vi "PD250 - PWM test_v2.vi"(8 "error in":errorcluster, 9 "Board Selector":T1, 10 "HMP VISA":refnum<visa-resource-name>, 11 "Control Board VISA":refnum<visa-resource-name>="ControlBoard") -> (0 "error out":errorcluster, 2 "Message OUT":string, 3 "Result (bool)":bool)   [LabVIEW 2022 SP3]
uses:
  Serial Board Com/Board Select.ctl
  HMP4000 Communication/HMP4040_ChannelControlAutomatic.ctl
  <vilib>/DAQmx/read.llb/DAQmx Read (Analog 1D Wfm NChan NSamp).vi
  <vilib>/DAQmx/miscellaneous.llb/DAQmx Fill In Error Info.vi
panel:
  out "Duty Cycle VISA Write":string[](array[string])
  out "ControlBoard OUT":refnum<visa-resource-name>
  in  "Message IN":string=" "
  out "Analysis Leg":i32
  out "Waveforms":T2
  out "Active Leg":i32
  out "Result (color)":u32(colorbox)
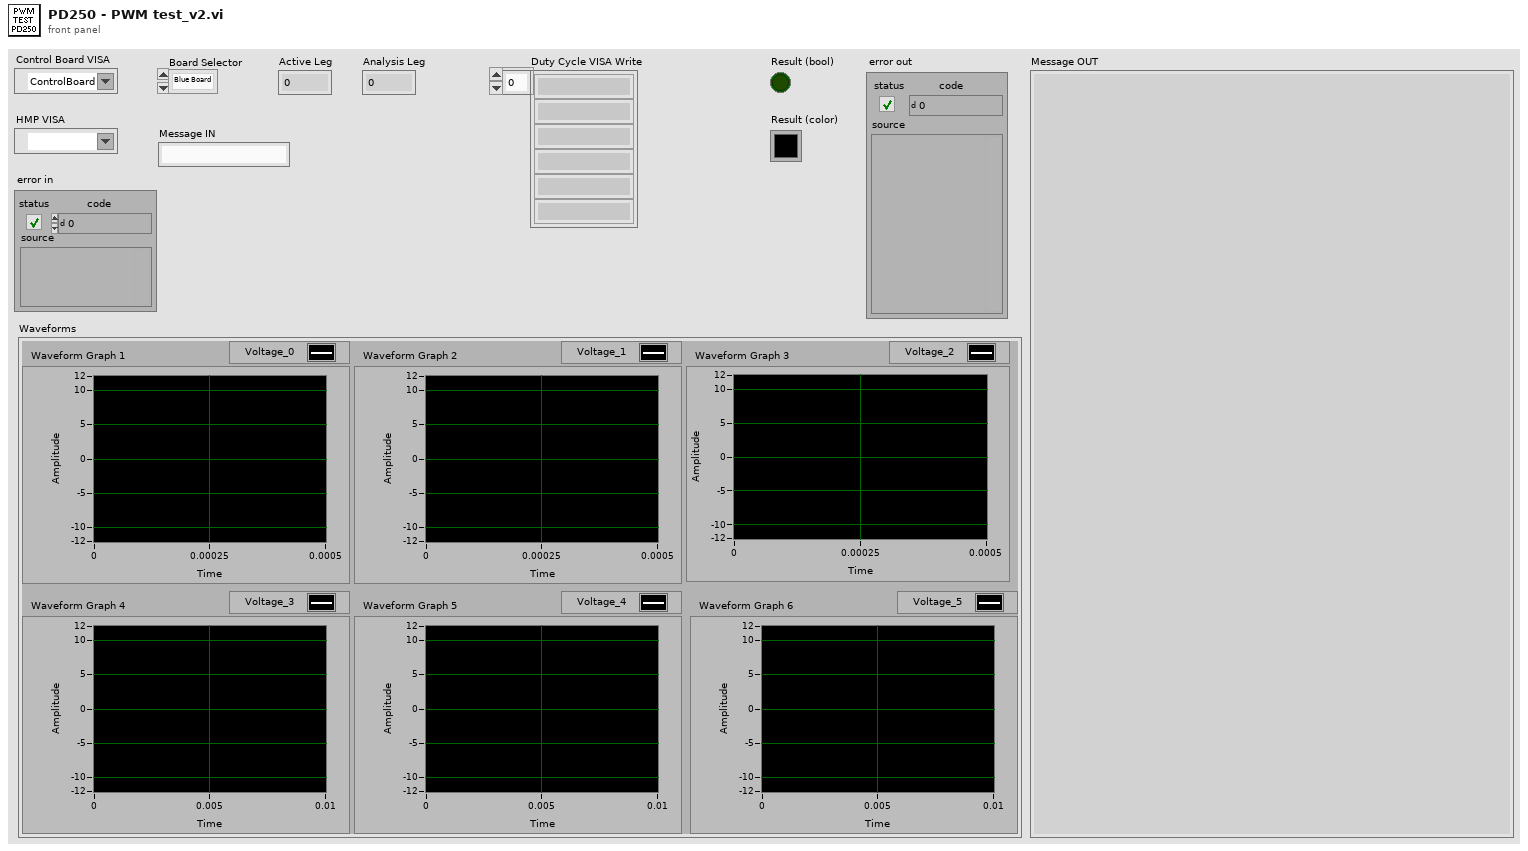
[diagram p1: front panel]
types:
  T1 = typedef "Board Select.ctl" = enum16{"Blue Board", "Green Board"}
  T2 = cluster{"Waveform Graph 1":waveform(dbl), "Waveform Graph 2":waveform(dbl), "Waveform Graph 3":waveform(dbl), "Waveform Graph 4":waveform(dbl), "Waveform Graph 5":waveform(dbl), "Waveform Graph 6":waveform(dbl)}
  T3 = typedef "HMP4040_ChannelControlAutomatic.ctl" = enum16{"Off", "Control Power", "HMP2020 Control + DC32V", "HMP2020 Control + DC8V", "HMP4040 Control + DC32V", "HMP4040 Control +DC8V", "HMP4040 Ch2 24V 4A"}
  T4 = cluster{"data[0]":waveform(dbl), "data[1]":waveform(dbl), "data[2]":waveform(dbl), "data[3]":waveform(dbl), "data[4]":waveform(dbl), "data[5]":waveform(dbl)}
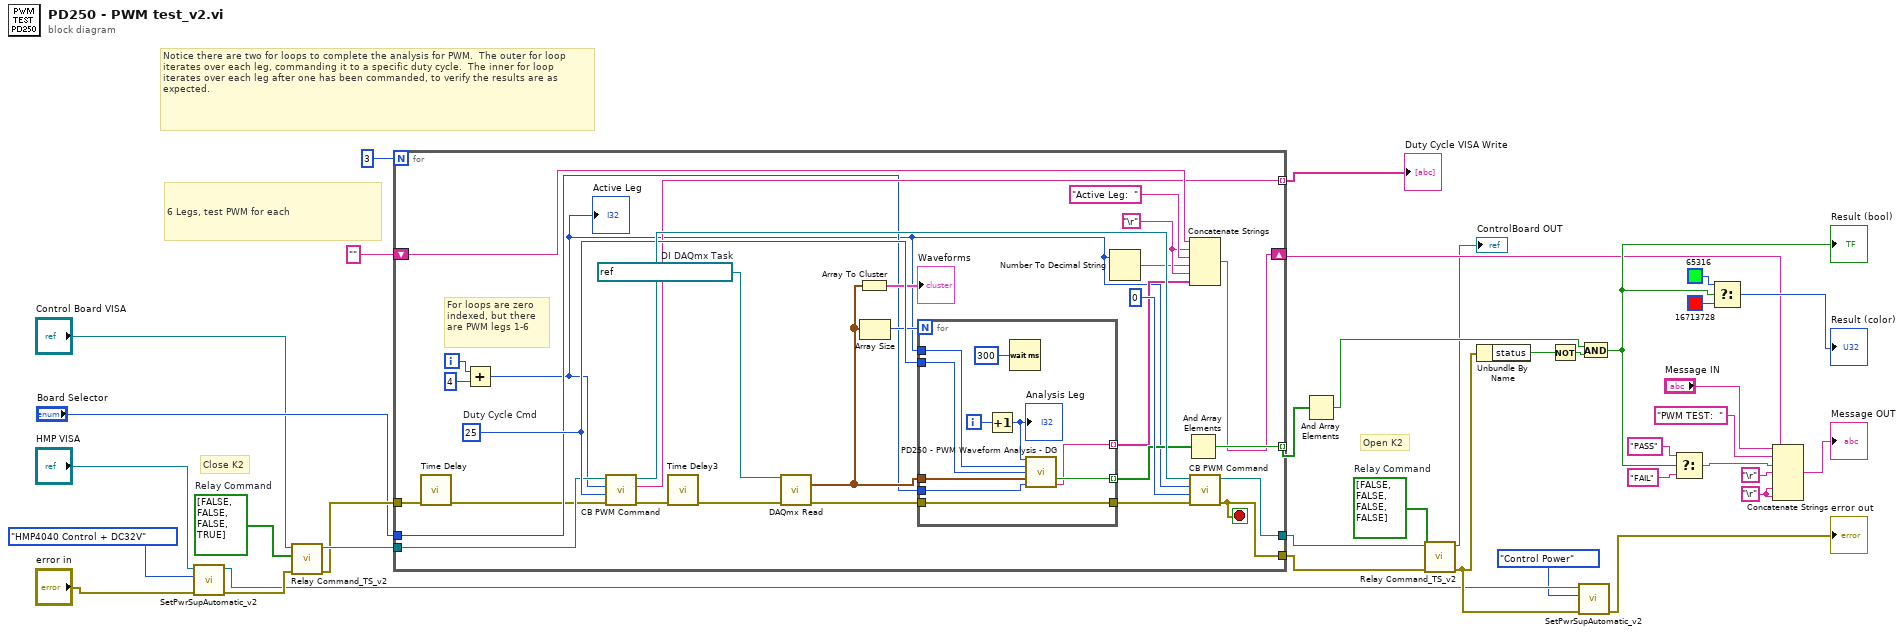
[diagram p0: block diagram]
diagram:
  w13 = bool[] [FALSE, FALSE, FALSE, TRUE]  # Relay Command
  w7 = bool[] [FALSE, FALSE, FALSE, FALSE]  # Relay Command
  w26 = "\r"
  # "Close K2"
  # "Open K2"
  # "Notice there are two for loops to complete the analysis for PWM.  The outer for loop iterates over each leg, commanding it to a specific duty cycle.  The inner for loop iterates over each leg after one has been commanded, to verify the results are as expected."
  # "6 Legs, test PWM for each"
  n1 = call "SetPwrSupAutomatic_v2.vi"("error in (no error)"="error in", "Enum"=HMP4040_ChannelControlAutomatic."HMP4040 Control + DC32V", "HMP VISA"="HMP VISA") -> ("error out"=w11:errorcluster, "HMP VISA Out"=w6:refnum<visa-resource-name>)  [unwired: 7 in]
  n2 = call "Relay Command_TS_v2.vi"("error in (no error)"=w11, "Relay Command"=w13, "Control Board VISA"="Control Board VISA") -> ("error out"=w15:errorcluster, "VISA Refnum out"=w16:refnum<visa-resource-name>)  [unwired: 7 in]
  n3 = for {
    N: 3 -> [_]
    tunnel: [w66] -> w37 mode=indexing
    shift-right: [w64] -> w24
    shift-left: "" -> [w63]
    tunnel: [w59] -> w18
    tunnel: [w54] -> w4
    tunnel: w15 -> [w44]
    tunnel: w16 -> [w49]
    tunnel: [w46] -> w14 mode=indexing
    tunnel: "Board Selector" -> [w45]
    i -> [w39]
    stop <- w59 stop-if-true
    w51 = "\r"
    w60 = 25  # Duty Cycle Cmd
    w65 = refnum<k21> "FTS2_PWMInput_DG"  # DI DAQmx Task
    # "For loops are zero indexed, but there are PWM legs 1-6"
    n4 = call "Time Delay"("error in (no error)"=w44) -> ("error out"=w43:errorcluster)  [unwired: 10 in]
    n5 = Add(x=w39, y=4) -> (x+y=w40:i32)
    "Active Leg" <- w40
    n6 = call "CB PWM Command.vi"("error in (no error)"=w43, "Duty Cycle"=w60, "Leg"=w40, "VISA Refnum in"=w49) -> ("error out"=w48:errorcluster, "read buffer"=w46:string, "VISA Refnum out"=w61:refnum<visa-resource-name>)  [unwired: 5 in]
    n7 = call "Time Delay3"("error in (no error)"=w48) -> ("error out"=w47:errorcluster)  [unwired: 10 in]
    n8 = call-poly <vilib>:"DAQmx Read.vi"("task/channels in"=w65, "error in"=w47) -> ("data"=w55:waveform(dbl)[], "error out"=w41:errorcluster)  [unwired: 11 in, 1 out]
    n9 = Array To Cluster(array=w55) -> (cluster=→"Waveforms":T4)
    n10 = Array Size(array=w55) -> (size(s)=w56:i32)
    n11 = for {
      N: w56 -> [_]
      tunnel: w60 -> [w76]
      tunnel: w55 -> [w75]
      tunnel: w40 -> [w74]
      tunnel: [w73] -> w57 mode=indexing
      tunnel: [w72] -> w52 mode=indexing
      tunnel: w45 -> [w71]
      tunnel: [w70] -> w42
      tunnel: w41 -> [w70]
      i -> [w68]
      n12 = Increment(x=w68) -> (x+1=w67:i32)
      "Analysis Leg" <- w67
      n13 = Wait (ms)(milliseconds to wait=u32 300) -> ()  [unwired: 1 out]
      n14 = call "PD250 - PWM Waveform Analysis - DG.vi"("Analysis Leg"=w67, "Active Leg"=w74, "Duty Cycle"=w76, "Waveform"=w75, "Board Selector"=w71) -> ("Result (Boolean)"=w73:bool, "Message"=w72:string)  [unwired: 9 in]
    }
    n15 = Number To Decimal String(number=w40) -> (decimal integer string=w50:string)  [unwired: 1 in]
    n16 = And Array Elements(Boolean array=w57) -> (logical AND=w66:bool)
    n17 = Concatenate Strings(w63, w51, "Active Leg:  ", w50, w51, w52) -> (w64:string)
    n18 = call "CB PWM Command.vi"("error in (no error)"=w42, "Duty Cycle"=0, "Leg"=w40, "VISA Refnum in"=w61) -> ("error out"=w59:errorcluster, "VISA Refnum out"=w54:refnum<visa-resource-name>)  [unwired: 5 in, 1 out]
  }
  "Duty Cycle VISA Write" <- w14
  n19 = And Array Elements(Boolean array=w37) -> (logical AND=w27:bool)
  n20 = call "Relay Command_TS_v2.vi"("error in (no error)"=w18, "Relay Command"=w7, "Control Board VISA"=w4) -> ("error out"=w10:errorcluster, "VISA Refnum out"=→"ControlBoard OUT":refnum<visa-resource-name>)  [unwired: 7 in]
  n21 = Unbundle By Name(w10) -> ("status"=w30:bool)
  n22 = Not(x=w30) -> (.not. x?=w29:bool)
  n23 = call "SetPwrSupAutomatic_v2.vi"("error in (no error)"=w10, "Enum"=HMP4040_ChannelControlAutomatic."Control Power", "HMP VISA"=w6) -> ("error out"=→"error out":errorcluster)  [unwired: 7 in, 1 out]
  n24 = And(x=w27, y=w29) -> (x .and. y?=w28:bool)
  "Result (bool)" <- w28
  n25 = Select(t="PASS", s=w28, f="FAIL") -> (s? t:f=w19:string)
  n26 = Select(t=u32 65316 ("Result (color)"), s=w28, f=u32 16713728 ("Result (color)")) -> (s? t:f=→"Result (color)":u32)
  n27 = Concatenate Strings("Message IN", "PWM TEST:  ", w19, "\r", w24, w26, w26) -> (→"Message OUT":string)
